vi "Dispense FN - OFF - State Status (SubVI).vi"(1 "Measured Mass (g)":dbl, 2 "Static Setpoint (g)":dbl, 3 "Timeout (s)":dbl, 4 "State Change Pulse":bool) -> (14 "Complete":bool, 15 "Timed Out":bool, 16 "Time Elapsed (s)":dbl)   [LabVIEW 2012]
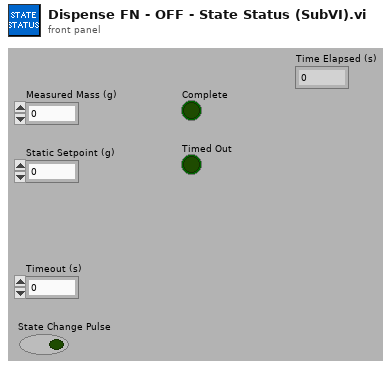
[diagram p1: front panel]
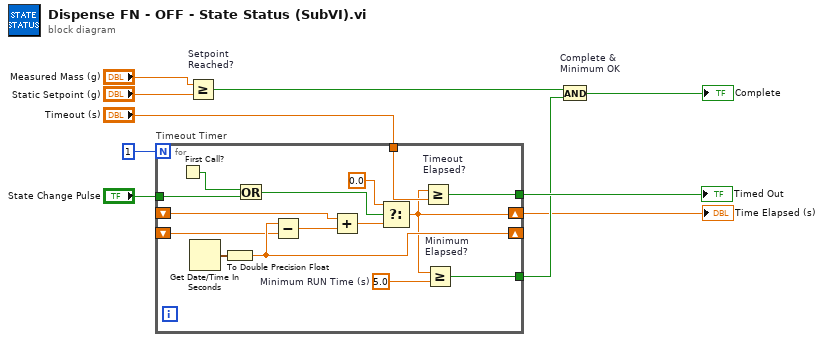
[diagram p0: block diagram]
diagram:
  n1 = for "Timeout Timer" {
    N: 1 -> [_]
    shift-right: [w15] -> w2
    shift-left: _ -> [w25]
    shift-right: [w21] -> _
    shift-left: _ -> [w20]
    tunnel: [w22] -> w8
    tunnel: "State Change Pulse" -> [w19]
    tunnel: "Timeout (s)" -> [w18]
    tunnel: [w13] -> w7
    w14 = 5.0  # Minimum RUN Time (s)
    n2 = First Call?() -> (First Call?: T/F=w16:bool)
    n3 = Get Date/Time In Seconds() -> (seconds since 1Jan1904=w24:timestamp)
    n4 = To Double Precision Float(number=w24) -> (double precision float=w21:dbl)
    n5 = Or(x=w16, y=w19) -> (x .or. y?=w12:bool)
    n6 = Subtract(x=w21, y=w20) -> (x-y=w17:dbl)
    n7 = Add(x=w25, y=w17) -> (x+y=w23:dbl)
    n8 = Select(t=0.0, s=w12, f=w23) -> (s? t:f=w15:dbl)
    n9 = Greater Or Equal? "Timeout\nElapsed?"(x=w15, y=w18) -> (x >= y?=w22:bool)
    n10 = Greater Or Equal? "Minimum\nElapsed?"(x=w15, y=w14) -> (x >= y?=w13:bool)
  }
  "Timed Out" <- w8
  "Time Elapsed (s)" <- w2
  n11 = Greater Or Equal? "Setpoint\nReached?"(x="Measured Mass (g)", y="Static Setpoint (g)") -> (x >= y?=w3:bool)
  n12 = And "Complete &\nMinimum OK"(x=w3, y=w7) -> (x .and. y?=→"Complete":bool)
